vi "SVT FFT Spectrum Subset (Real-Im) (1 Ch).vi"(0 "scaled signal [EU]":waveform(dbl)={"t0"=timestamp(0 s since 1904-01-01), "dt"=1e-05, "Y"=[]}, 2 "window":T8=1 items=["None"=0, "Hanning"=1, "Hamming"=2, "Blackman-Harris"=3, "Exact Blackman"=4, "Blackman"=5, "Flat Top"=6, "4 Term B-Harris "=7, "7 Term B-Harris"=8, "Low Sidelobe"=9, "Blackman Nuttall"=11, "Triangle"=30, "Bartlett-Hanning"=31, "Bohman"=32, "Parzen"=33, "Welch"=34, "Kaiser"=60, "Dolph-Chebyshev"=61, "Gaussian"=62], 3 "frequency range":T10={"start frequency"=1000.0, "stop frequency"=5000.0} {"stop frequency" min=0.0 format="%.2f"; "start frequency" min=0.0 format="%.2f"}, 5 "error in (no error)":errorcluster, 7 "averaging parameters":T9={"averaging mode"=enum."No averaging", "weighting mode"=enum."Exponential", "number of averages"=10, "linear mode"=enum."One shot"} {"number of averages" min=1 step=1}, 9 "restart averaging (F)":bool) -> (11 "averaging done":bool, 13 "averages completed":dbl=1.0, 14 "real part [EU rms]":cluster{"f0":dbl, "df":dbl, "real part":dbl[]}={"f0"=nan, "df"=inf, "real part"=[]} {"real part" format="%.2f"; "df" format="%.2f"; "f0" format="%.2f"}, 16 "imaginary part [EU rms]":T1={"f0"=nan, "df"=inf, "imaginary part"=[]} {"imaginary part" format="%.2f"; "df" format="%.2f"; "f0" format="%.2f"}, 17 "unit label":string, 18 "spectrum info":T2={"channel name"="", "description"="", "x-axis units"=1, "spectral info"={"spectrum type"=enum."Power [Magnitude^2]", "linear/dB"=enum."linear", "window"=0, "window size"=0, "FFT size"=0}, "engineering units"=0, "custom label"="", "dB reference [EU]"=0.0, "peak units"=enum."rms", "weighting filter"=0, "spectral density?"=FALSE, "unit label"="", "spectrum skewed?"=FALSE, "complimentary spectrum units"=enum."none"} {"x-axis units" items=["Time (s)"=0, "Frequency-CB (Hz)"=1, "Frequency-CPB (Hz)"=1248, "Frequency-Arbitrary (Hz)"=2357, "Quefrency (s)"=2, "Revolutions (rev)"=3, "Order"=4, "Speed (RPM)"=11, "Speed (rad/s)"=21, "Index"=65535]; "weighting filter" items=["Linear", "A-weighting", "B-weighting", "C-weighting", "ITU-R 468-4", "Dolby", "CCITT", "C-message", "Wb", "Wc", "Wd", "We", "Wf", "Wh", "Wj", "Wk", "Wm", "AES17 20 kHz lowpass", "AES17 40 kHz lowpass", "AES17 20 kHz highpass", "AES17 40 kHz highpass"]; "dB reference [EU]" format="%.2f"; "engineering units" items=["custom..."=0, "V"=1, "A"=21, "C"=30, "pC"=31, "s"=32, "-"=29, "Pa"=2, "N"=20, "g"=3, "m/s^2"=4, "m/s"=5, "m"=6, "mm/s"=12, "mm"=13, "micron/s"=14, "micron"=15, "in/s^2"=7, "in/s"=8, "in"=9, "mil/s"=10, "mil"=11, "rad/s^2"=16, "rad/s"=17, "rad"=18, "deg/s^2"=26, "deg/s"=27, "deg"=28, "RPM"=22, "cycle/s^2"=23, "Hz"=24, "cycle"=25, "strain"=19]; "spectral info"."window" items=["None "=0, "Hanning"=1, "Hamming"=2, "Blackman-Harris"=3, "Exact Blackman"=4, "Blackman"=5, "Flat Top"=6, "4 Term B-Harris "=7, "7 Term B-Harris"=8, "Low Sidelobe"=9, "Force - Exponential"=10, "Gaussian"=62]}, 19 "error out":errorcluster)   [LabVIEW 2017]
doc: "Computes a subset of the FFT spectrum of <B>scaled signal [EU]</B>. The subset is defined by <B>frequency range</B>. FFT results are returned as <B>real part [EU rms]</B> and <B>imaginary part [EU rms]</B>. Each block of data corresponds to a single FFT block and has to be passed individually to the this VI. You can use this polymorphic VI to analyze signals from a single channel or from N channels. The data type you wire to the <B>scaled signal [EU]</B> input determines the polymorphic instance to use."
uses:
  <vilib>/addons/_NISVFA/_Shared subVIs/Controls/svc_Window.ctl
  <vilib>/addons/_NISVFA/_Shared subVIs/Controls/svc_Spectrum Info.ctl
  <vilib>/addons/_NISVFA/_Shared subVIs/Controls/svc_X-Axis Units.ctl
  <vilib>/addons/_NISVFA/_Shared subVIs/Controls/svc_Spectrum Type.ctl
  <vilib>/addons/_NISVFA/_Shared subVIs/Controls/svc_Engineering Units Text Ring.ctl
  <vilib>/addons/_NISVFA/_Shared subVIs/Controls/svc_Weighting Filter Text Ring.ctl
  <vilib>/addons/_NISVFA/_Shared subVIs/Controls/svc_Complimentary Spectrum Units.ctl
  <vilib>/addons/_NISVFA/_Shared subVIs/Windowing/svfa_Scaled Time Domain Window (Array).vi
  <vilib>/addons/_NISVFA/_Shared subVIs/Common/svc_Get SV Channel Info.vi
  <vilib>/addons/_NISVFA/_Shared subVIs/Common/svc_Spectrum Units.vi
  <vilib>/addons/_NISVFA/_Shared subVIs/Spectrum Averaging/svfa_Reset Averaging State Info.vi
  <vilib>/addons/_NISVFA/_Shared subVIs/Spectrum Averaging/svfa_Average Array with Avg Checks (complex) No State.vi
  <vilib>/addons/_NISVFA/_Shared subVIs/Common/svc_Complex to Mag2 Array.vi
  <vilib>/addons/_NISVFA/_Shared subVIs/Spectrum Averaging/svfa_Average Array with Avg Checks (real) No State.vi
  <vilib>/Analysis/4window.llb/Force Window.vi
  <vilib>/Analysis/4window.llb/Force Window (DBL).vi
  <vilib>/Analysis/4window.llb/Exponential Window.vi
  <vilib>/Analysis/4window.llb/Exponential Window (DBL).vi
  <vilib>/addons/_NISVFA/_Shared subVIs/Spectrum Averaging/svfa_Average Array (complex) No State.vi
  <vilib>/addons/_NISVFA/_Shared subVIs/Spectrum Averaging/svfa_Average Array (real) No State.vi
  <vilib>/addons/_NISVFA/_Shared subVIs/Spectrum Averaging/svfa_No Average Array (complex).vi
  <vilib>/addons/_NISVFA/_Shared subVIs/Spectrum Averaging/svfa_Average Array (complex).vi
  <vilib>/addons/_NISVFA/_Shared subVIs/Spectrum Averaging/svfa_No Average Array (real).vi
  <vilib>/addons/_NISVFA/_Shared subVIs/Spectrum Averaging/svfa_Average Array (real).vi
  <vilib>/addons/_NISVFA/_Shared subVIs/Spectrum Averaging/svfa_Peak Hold Array.vi
  <vilib>/addons/_NISVFA/_Shared subVIs/Common/svc_Get Weighting Enum and Labels.vi
  <vilib>/addons/_NISVFA/_Shared subVIs/Common/svc_Unit Label Lexical Class.vi
  <vilib>/addons/_NISVFA/_Shared subVIs/Common/svc_Engineering Units to Unit Label.vi
  <vilib>/addons/_NISVFA/_Shared subVIs/Common/svc_Format Value (DBL).vi
  <vilib>/addons/_NISVFA/_Shared subVIs/Common/svc_Channel Info to Spectrum Info.vi
  <vilib>/addons/_NISVFA/_Shared subVIs/Common/svc_Unit Label to Engineering Units.vi
  <vilib>/Utility/error.llb/Error Cluster From Error Code.vi
  <vilib>/Analysis/0measdsp.llb/Scaled Time Domain Window.vi
  <vilib>/Analysis/0measdsp.llb/Scaled Time Domain Window (DBL).vi
  <vilib>/addons/_NISVFA/_Spectrum Processing/subVIs/svfa_Spectrum Info Window to windowTd Type Def.vi
  <vilib>/addons/_NISVFA/_Shared subVIs/Common/svc_Window Parameters.vi
  <vilib>/addons/_NISVFA/_Shared subVIs/Common/svc_Get Window Info.vi
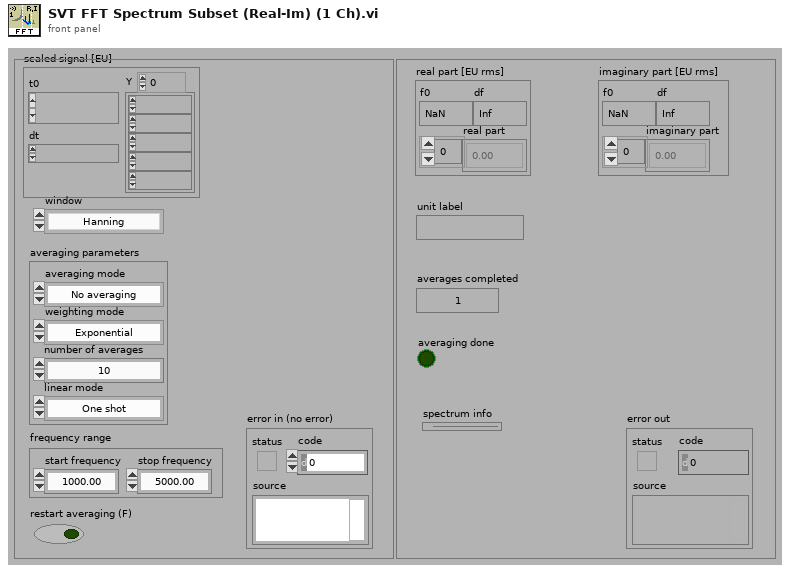
[diagram p1: front panel]
types:
  T1 = cluster{"f0":dbl, "df":dbl, "imaginary part":dbl[]}
  T2 = typedef "svc_Spectrum Info.ctl" = cluster{"channel name":string, "description":string, "x-axis units":T3, "spectral info":cluster{"spectrum type":T4, "linear/dB":enum16{"linear", "dB"}, "window":u16, "window size":i32, "FFT size":i32}, "engineering units":T5, "custom label":string, "dB reference [EU]":dbl, "peak units":enum16{"rms", "peak", "peak-peak"}, "weighting filter":T6, "spectral density?":bool, "unit label":string, "spectrum skewed?":bool, "complimentary spectrum units":T7}
  T3 = typedef "svc_X-Axis Units.ctl" = u16
  T4 = typedef "svc_Spectrum Type.ctl" = enum16{"FFT Spectrum [complex]", "Amplitude [Magnitude]", "Power [Magnitude^2]", "Cross Spectrum [complex]", "Frequency Response [Complex]"}
  T5 = typedef "svc_Engineering Units Text Ring.ctl" = u16
  T6 = typedef "svc_Weighting Filter Text Ring.ctl" = u16
  T7 = typedef "svc_Complimentary Spectrum Units.ctl" = enum16{"none", "radians", "degrees", "cycles", "imaginary"}
  T8 = typedef "svc_Window.ctl" = u32
  T9 = cluster{"averaging mode":enum16{"No averaging", "Vector averaging", "RMS averaging", "Peak hold"}, "weighting mode":enum16{"Linear", "Exponential"}, "number of averages":u32, "linear mode":enum16{"One shot", "Auto restart"}}
  T10 = cluster{"start frequency":dbl, "stop frequency":dbl}
  T11 = cluster{"f0":dbl, "df":dbl, "complex spectrum":cdb[]}
  T12 = enum16{"Restart processing", "Continue processing", "Skip processing"}
  T13 = enum16{"No averaging", "Vector averaging", "RMS averaging", "Peak hold"}
  T14 = cluster{"complex FFT":cdb[], "real FFT":dbl[], "f0":dbl, "df":dbl, "averages completed":dbl, "averaging parameters":cluster{"averaging mode":enum16{"No averaging", "Vector averaging", "RMS averaging", "Peak hold"}, "weighting mode":enum16{"Linear", "Exponential"}, "number of averages":u32, "linear mode":enum16{"One shot", "Auto restart"}}}
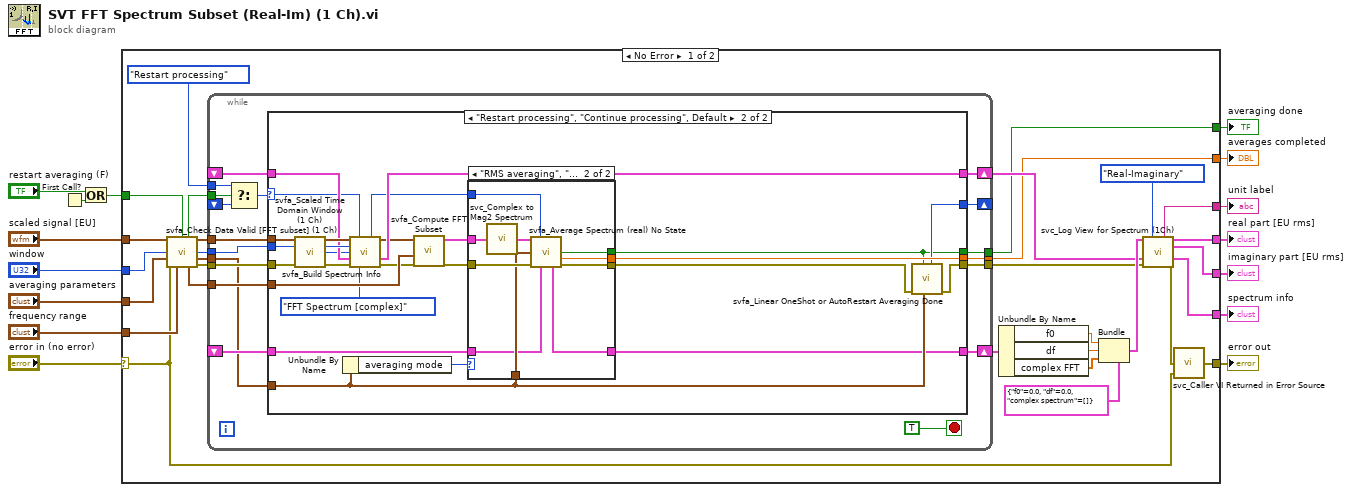
[diagram p0: block diagram]
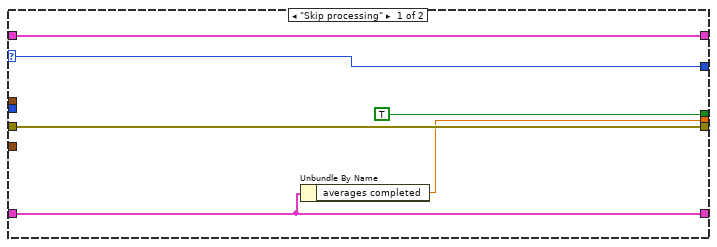
[diagram p2: hidden frame]
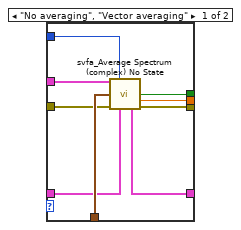
[diagram p3: hidden frame]
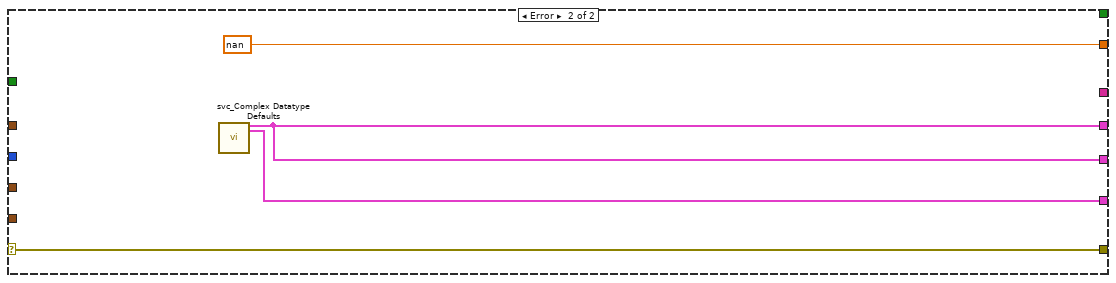
[diagram p4: hidden frame]
diagram:
  n1 = First Call?() -> (First Call?: T/F=w3:bool)
  n2 = Or(x="restart averaging (F)", y=w3) -> (x .or. y?=w1:bool)
  n3 = case shown="No Error" "error in (no error)" {
    selector: "error in (no error)" -> [w23 w118]
    tunnel: w1 -> [w24 _]
    tunnel: [w17 nan ("Averaged So-far")] -> w10
    tunnel: [w16 _] -> w8
    tunnel: [w22 w118] -> w9
    tunnel: "averaging parameters" -> [w25 _]
    tunnel: "frequency range" -> [w28 _]
    tunnel: "scaled signal [EU]" -> [w27 _]
    tunnel: "window" -> [w26 _]
    tunnel: [w19 w116] -> w7
    tunnel: [w18 _] -> w4
    tunnel: [w21 w115] -> w5
    tunnel: [w20 w115] -> w6
    frame No Error {
      n4 = call <vilib>:"svfa_Check Data Valid [FFT subset] (1 Ch).vi"("signal"=w27, "restart averaging (F)"=w24, "window"=w26, "averaging parameters"=w25, "error in (no error)"=w23, "frequency range in"=w28) -> ("restart averaging"=w34:bool, "dup signal"=w39:waveform(dbl), "window"=w38:u16, "dup averaging parameters"=w35:T9, "frequency range out"=w37:T10, "error out"=w36:errorcluster)  [unwired: 4 in]
      n5 = while {
        shift-left: _ -> [w55]
        shift-right: [w56] -> w40
        tunnel: w37 -> [w58]
        tunnel: w39 -> [w59]
        tunnel: [w60] -> w17
        tunnel: [w62] -> w16
        tunnel: w36 -> [w63]
        tunnel: [w61] -> w31
        tunnel: w38 -> [w51]
        shift-right: [w53] -> w30
        shift-left: _ -> [w52]
        tunnel: w35 -> [w50]
        tunnel: w34 -> [w49]
        shift-right: [w57] -> _
        shift-left: _ -> [w48]
        tunnel: T12."Restart processing" ("processing control") -> [w47]
        stop <- TRUE stop-if-true
        n6 = Select(t=w47, s=w49, f=w48) -> (s? t:f=w46:T12)
        n7 = case shown="\"Restart processing\", \"Continue processing\", Default" w46 {
          selector: w46 -> [w67 w70]
          tunnel: w50 -> [_ w91]
          tunnel: [w66 w85] -> w56
          tunnel: w59 -> [_ w94]
          tunnel: w58 -> [_ w78]
          tunnel: [w67 w90] -> w57
          tunnel: w55 -> [w66 w84]
          tunnel: w51 -> [_ w92]
          tunnel: [w64 w75] -> w53
          tunnel: w52 -> [w64 w76]
          tunnel: [TRUE ("averaging done?") w87] -> w62
          tunnel: [w65 w95] -> w60
          tunnel: [w68 w89] -> w61
          tunnel: w63 -> [w68 w93]
          frame "Skip processing" {
            n8 = Unbundle By Name(w66) -> ("averages completed"=w65:dbl)
          }
          frame "Restart processing", "Continue processing", Default {
            n9 = call <vilib>:"svfa_Scaled Time Domain Window (1 Ch).vi"("Signal in [X]"=w94, "window"=w92, "error in"=w93) -> ("Windowed Waveform"=w81:waveform(dbl), "dup window"=w82:T8, "window length"=w72:i32, "error out"=w83:errorcluster)  [unwired: 7 in, 2 out]
            n10 = Unbundle By Name(w91) -> ("averaging mode"=w86:T13)
            n11 = call <vilib>:"svfa_Build Spectrum Info.vi"("scaled signal [EU]"=w81, "processing control"=w70, "window"=w82, "window size"=w72, "spectrum info in"=w76, "error in (no error)"=w83, "spectrum type"=svc_Spectrum_Type."FFT Spectrum [complex]" ("spectrum type 2")) -> ("dup processing control"=w74:T12, "dup scaled signal [EU]"=w71:waveform(dbl), "spectrum info out"=w75:T2, "error out"=w73:errorcluster)  [unwired: 5 in]
            n12 = call <vilib>:"svfa_Compute FFT Subset.vi"("error in (no error)"=w73, "frequency range"=w78, "windowed signal"=w71) -> ("error out"=w80:errorcluster, "FFT spectrum [Vrms]"=w79:cluster{"f0":dbl, "df":dbl, "spectrum":cdb[]})  [unwired: 7 in]
            n13 = case shown="\"RMS averaging\", \"Peak hold\"" w86 {
              tunnel: w91 -> [w103 w111]
              tunnel: [w101 w107] -> w88
              tunnel: [w100 w113] -> w87
              tunnel: w79 -> [w104 w108]
              tunnel: w80 -> [w102 w114]
              tunnel: [w98 w112] -> w95
              tunnel: w74 -> [w99 w109]
              tunnel: [w97 w105] -> w85
              tunnel: w84 -> [w96 w106]
              frame "No averaging", "Vector averaging" {
                n14 = call <vilib>:"svfa_Average Spectrum (complex) No State.vi"("spectrum"=w104, "processing control"=w99, "averaging parameters"=w103, "error in (no error)"=w102, "averaging state info in"=w96) -> ("averaging done"=w100:bool, "averages completed"=w98:dbl, "averaging state info out"=w97:T14, "error out"=w101:errorcluster)  [unwired: 5 in, 2 out]
              }
              frame "RMS averaging", "Peak hold" {
                n15 = call <vilib>:"svc_Complex to Mag2 Spectrum.vi"("complex spectrum"=w108) -> ("power spectrum"=w110:cluster{"f0":dbl, "df":dbl, "spectrum":dbl[]})  [unwired: 4 in]
                n16 = call <vilib>:"svfa_Average Spectrum (real) No State.vi"("spectrum"=w110, "processing control"=w109, "averaging parameters"=w111, "error in (no error)"=w114, "averaging state info in"=w106) -> ("averaging done"=w113:bool, "averages completed"=w112:dbl, "averaging state info out"=w105:T14, "error out"=w107:errorcluster)  [unwired: 5 in, 2 out]
              }
            }
            n17 = call <vilib>:"svfa_Linear OneShot or AutoRestart Averaging Done.vi"("averaging parameters"=w91, "averaging done"=w87, "error in (no error)"=w88) -> ("error out"=w89:errorcluster, "processing control"=w90:T12)  [unwired: 7 in]
          }
        }
      }
      n18 = Unbundle By Name(w40) -> ("f0"=w43:dbl, "df"=w42:dbl, "complex FFT"=w41:cdb[])
      n19 = Bundle(cluster=T11 {"f0"=0.0, "df"=0.0, "complex spectrum"=[]} ("complex spectrum response"), "f0"=w43, "df"=w42, "complex spectrum"=w41) -> (w32:T11)
      n20 = call <vilib>:"svc_Log View for Spectrum (1Ch).vi"("complex spectrum"=w32, "View"=enum16{"Mag-Phase", "Real-Imaginary"}."Real-Imaginary", "spectrum info in"=w30, "error in (no error)"=w31) -> ("unit label [mag or real]"=w18:string, "magnitude or real"=w21:cluster{"f0":dbl, "df":dbl, dbl[]}, "phase or imag"=w20:cluster{"f0":dbl, "df":dbl, dbl[]}, "spectrum info out"=w19:T2, "error out"=w45:errorcluster)  [unwired: 6 in, 1 out]
      n21 = call <vilib>:"svc_Caller VI Returned in Error Source.vi"("warning input to caller"=w23, "error in (no error)"=w45) -> ("error out"=w22:errorcluster)  [unwired: 3 in]
    }
    frame Error {
      n22 = call <vilib>:"svc_Complex Datatype Defaults.vi"() -> ("empty spectrum"=w115:cluster{"f0":dbl, "df":dbl, "magnitude":dbl[]}, "dead spectrum info"=w116:T2)  [unwired: 11 in, 7 out]
    }
  }
  "averages completed" <- w10
  "averaging done" <- w8
  "error out" <- w9
  "spectrum info" <- w7
  "unit label" <- w4
  "real part [EU rms]" <- w5
  "imaginary part [EU rms]" <- w6
